vi "LVClass_Image get image data.vi"(0 "Image in":refnum<class "Image.lvclass">, 11 "error in (no error)":errorcluster) -> (4 "Image out":refnum<class "Image.lvclass">, 6 "Image data out":u32[][](array[numeric]), 15 "error out":errorcluster)   [LabVIEW 2020, in "Image.lvclass"]
uses:
  Image.lvclass
  Point2D.ctl
  LVClass_Image Read Image.vi
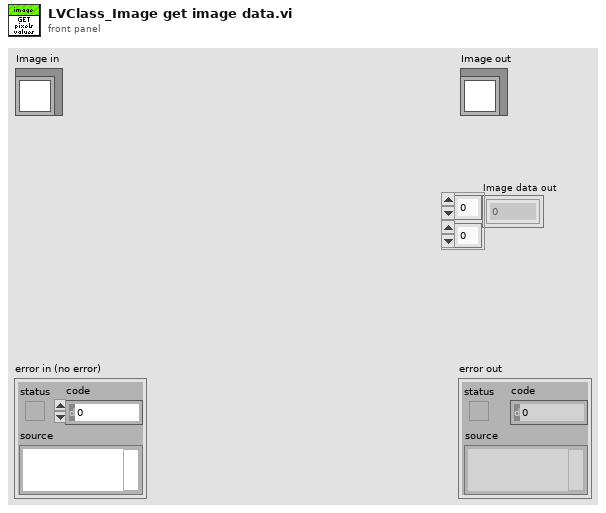
[diagram p1: front panel]
types:
  T1 = typedef "Point2D.ctl" = cluster{"X":u32, "Y":u32}
  T2 = typedef "Data alignment enum.ctl" = enum16{"8", "16", "32"}
  T3 = typedef "Struct_Image.ctl" = cluster{"Image_Handler":T4, "Number of bits":T2, "ImageSize":T1}
  T4 = typedef "ClassID.ctl" = i64
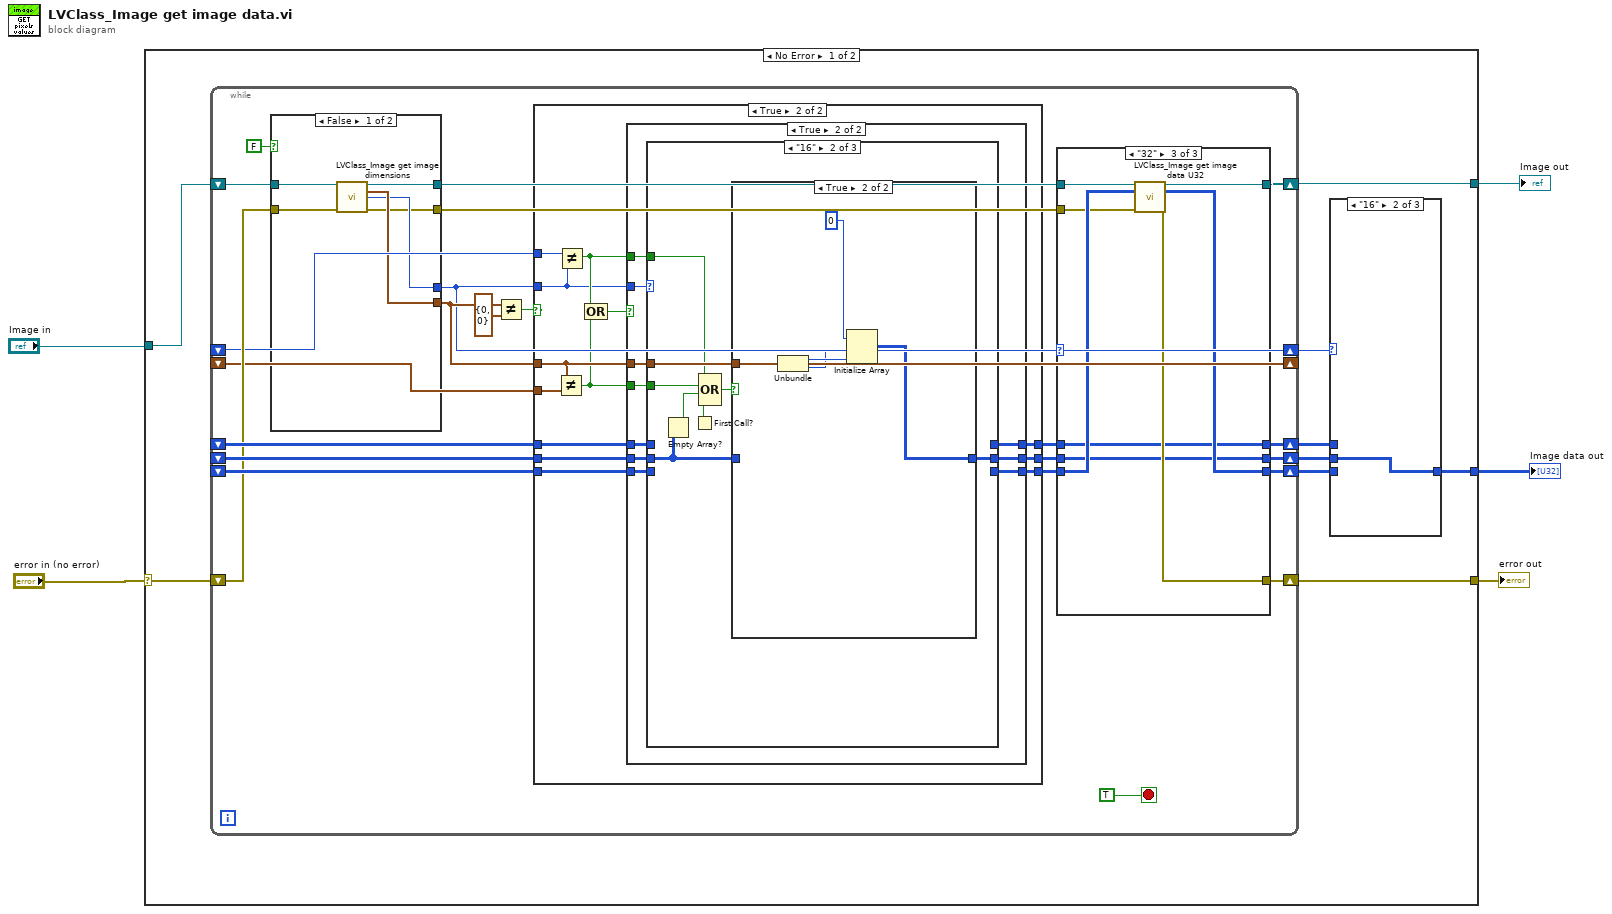
[diagram p0: block diagram]
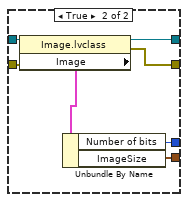
[diagram p4: hidden frame]
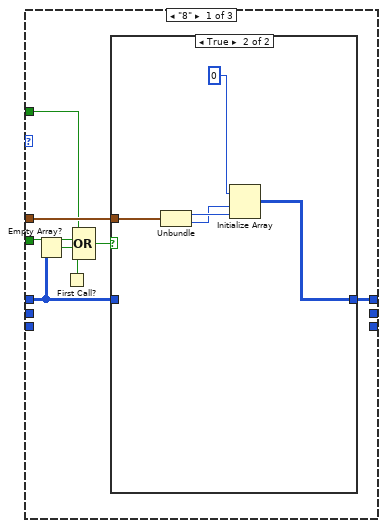
[diagram p7: hidden frame]
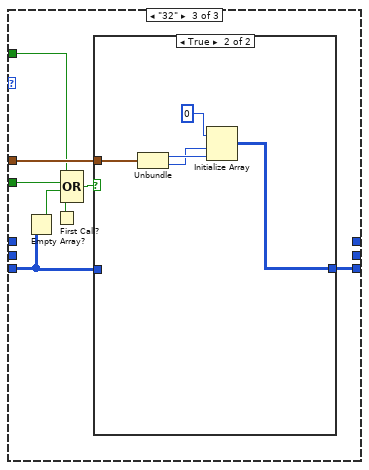
[diagram p10: hidden frame]
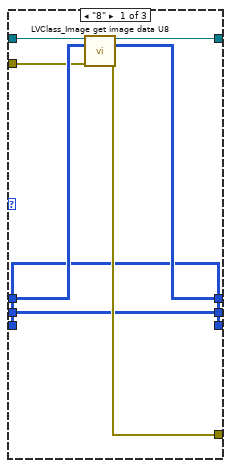
[diagram p12: hidden frame]
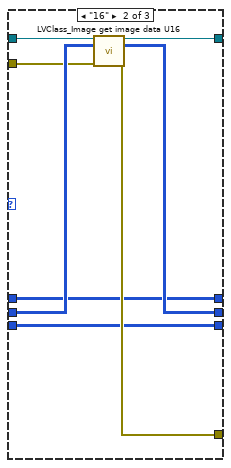
[diagram p13: hidden frame]
diagram:
  n1 = case shown="No Error" "error in (no error)" {
    selector: "error in (no error)" -> [w12 w150]
    tunnel: [w11 w150] -> w4
    tunnel: [w14 w149] -> w2
    tunnel: "Image in" -> [w13 w149]
    tunnel: [w8 _] -> w1
    frame No Error {
      n2 = while {
        shift-right: [w39] -> w9
        shift-left: _ -> [w36]
        shift-right: [w38] -> w7
        shift-left: _ -> [w35]
        shift-right: [w40] -> w6
        shift-left: _ -> [w34]
        shift-right: [w33] -> w14
        shift-left: w13 -> [w30]
        shift-right: [w32] -> w11
        shift-left: w12 -> [w29]
        shift-right: [w27] -> _
        shift-left: _ -> [w19]
        shift-right: [w20] -> w10
        shift-left: _ -> [w21]
        stop <- TRUE stop-if-true
        n3 = case shown="False" FALSE {
          tunnel: [w44 w53] -> w31
          tunnel: w30 -> [w43 w52]
          tunnel: w29 -> [w42 w51]
          tunnel: [w46 w50] -> w27
          tunnel: [w41 w48] -> w26
          tunnel: [w45 w47] -> w20
          frame False {
            n4 = call "LVClass_Image get image dimensions.vi"("Image in"=w43, "error in (no error)"=w42) -> ("Image out"=w44:refnum<class "Image.lvclass">, "Number of pixels"=w46:T1, "Number of bits"=w45:T2, "error out"=w41:errorcluster)  [unwired: 10 in]
          }
          frame True {
            n5 = property class="Image.lvclass"(reference=w52, error in=w51) -> (reference out=w53:refnum<class "Image.lvclass">, error out=w48:errorcluster, "Image"=w49:T3)
            n6 = Unbundle By Name(w49) -> ("Number of bits"=w47:T2, "ImageSize"=w50:T1)
          }
        }
        n7 = Not Equal?(x=w27, y=T1 {"X"=0, "Y"=0}) -> (x != y?=w22:bool)
        n8 = case shown="True" w22 {
          tunnel: [w56 w69] -> w25
          tunnel: [w55 w68] -> w24
          tunnel: [w54 w67] -> w23
          tunnel: w36 -> [w56 w66]
          tunnel: w35 -> [w55 w65]
          tunnel: w34 -> [w54 w64]
          tunnel: w27 -> [_ w60]
          tunnel: w21 -> [_ w62]
          tunnel: w20 -> [_ w57]
          tunnel: w19 -> [_ w59]
          frame False {
          }
          frame True {
            n9 = Not Equal?(x=w60, y=w59) -> (x != y?=w58:bool)
            n10 = Not Equal?(x=w62, y=w57) -> (x != y?=w61:bool)
            n11 = Compound Arithmetic op=OR(w61, w58) -> (w63:bool)
            n12 = case shown="True" w63 {
              tunnel: [w72 w82] -> w69
              tunnel: [w71 w81] -> w68
              tunnel: [w70 w80] -> w67
              tunnel: w66 -> [w72 w79]
              tunnel: w65 -> [w71 w78]
              tunnel: w64 -> [w70 w77]
              tunnel: w60 -> [_ w76]
              tunnel: w57 -> [_ w75]
              tunnel: w58 -> [_ w74]
              tunnel: w61 -> [_ w73]
              frame False {
              }
              frame True {
                n13 = case shown="\"16\"" w75 {
                  tunnel: [w90 _ _] -> w82
                  tunnel: [_ w101 _] -> w81
                  tunnel: [_ _ w115] -> w80
                  tunnel: w79 -> [w85 _ _]
                  tunnel: w78 -> [_ w100 _]
                  tunnel: w77 -> [_ _ w114]
                  tunnel: w76 -> [w89 w104 w118]
                  tunnel: w74 -> [w83 w98 w112]
                  tunnel: w73 -> [w84 w99 w113]
                  frame "8" {
                    n14 = Empty Array?(array=w85) -> (empty?=w88:bool)
                    n15 = First Call?() -> (First Call?: T/F=w86:bool)
                    n16 = Compound Arithmetic op=OR(w84, w83, w88, w86) -> (w87:bool)
                    n17 = case shown="True" w87 {
                      tunnel: [w91 w96] -> w90
                      tunnel: w89 -> [_ w95]
                      tunnel: w85 -> [w91 _]
                      frame False {
                      }
                      frame True {
                        n18 = Unbundle(w95) -> ("X"=w94:u32, "Y"=w93:u32)
                        n19 = Initialize Array(u8 0 ("element"), w93, w94) -> (w96:u8[][])
                      }
                    }
                  }
                  frame "16" {
                    n20 = Empty Array?(array=w100) -> (empty?=w97:bool)
                    n21 = First Call?() -> (First Call?: T/F=w102:bool)
                    n22 = Compound Arithmetic op=OR(w99, w98, w97, w102) -> (w103:bool)
                    n23 = case shown="True" w103 {
                      tunnel: w104 -> [_ w110]
                      tunnel: [w105 w106] -> w101
                      tunnel: w100 -> [w105 _]
                      frame False {
                      }
                      frame True {
                        n24 = Unbundle(w110) -> ("X"=w109:u32, "Y"=w108:u32)
                        n25 = Initialize Array(u16 0 ("element"), w108, w109) -> (w106:u16[][])
                      }
                    }
                  }
                  frame "32" {
                    n26 = Empty Array?(array=w114) -> (empty?=w111:bool)
                    n27 = First Call?() -> (First Call?: T/F=w116:bool)
                    n28 = Compound Arithmetic op=OR(w113, w112, w111, w116) -> (w117:bool)
                    n29 = case shown="True" w117 {
                      tunnel: w118 -> [_ w124]
                      tunnel: [w119 w120] -> w115
                      tunnel: w114 -> [w119 _]
                      frame False {
                      }
                      frame True {
                        n30 = Unbundle(w124) -> ("X"=w123:u32, "Y"=w122:u32)
                        n31 = Initialize Array(u32 0 ("element"), w122, w123) -> (w120:u32[][])
                      }
                    }
                  }
                }
              }
            }
          }
        }
        n32 = case shown="\"32\"" w20 {
          tunnel: w31 -> [w128 w136 w143]
          tunnel: [w125 w133 w148] -> w40
          tunnel: [w132 w140 w147] -> w32
          tunnel: w25 -> [w131 w137 w145]
          tunnel: w24 -> [w129 w139 w144]
          tunnel: w23 -> [w125 w133 w146]
          tunnel: [w130 w137 w145] -> w39
          tunnel: [w129 w138 w144] -> w38
          tunnel: [w127 w135 w142] -> w33
          tunnel: w26 -> [w126 w134 w141]
          frame "8" {
            n33 = call "LVClass_Image get image data U8.vi"("Image in"=w128, "Image data"=w131, "error in (no error)"=w126) -> ("Image out"=w127:refnum<class "Image.lvclass">, "Image data out"=w130:u8[][], "error out"=w132:errorcluster)  [unwired: 10 in]
          }
          frame "16" {
            n34 = call "LVClass_Image get image data U16.vi"("Image in"=w136, "Image data"=w139, "error in (no error)"=w134) -> ("Image out"=w135:refnum<class "Image.lvclass">, "Image data out"=w138:u16[][], "error out"=w140:errorcluster)  [unwired: 10 in]
          }
          frame "32" {
            n35 = call "LVClass_Image get image data U32.vi"("Image in"=w143, "Image data"=w146, "error in (no error)"=w141) -> ("Image out"=w142:refnum<class "Image.lvclass">, "Image data out"=w148:u32[][], "error out"=w147:errorcluster)  [unwired: 10 in]
          }
        }
      }
      n36 = case shown="\"16\"" w10 {
        tunnel: w9 -> [w15 _ _]
        tunnel: [w15 w16 w17] -> w8
        tunnel: w7 -> [_ w16 _]
        tunnel: w6 -> [_ _ w17]
        frame "8", Default {
        }
        frame "16" {
        }
        frame "32" {
        }
      }
    }
    frame Error {
    }
  }
  "error out" <- w4
  "Image out" <- w2
  "Image data out" <- w1
